vi "Extract Video Moments.vi"() -> ()   [LabVIEW 2026]
uses:
  90f86d5b-f17d-465b-a039-599a13c3f885.vi
panel:
  out "Web Browser Control":string(html)
  out "appended array":cluster{"output 7":dbl, "Instruction":string}[](array[cluster])
  in  "Video to Inject":path=path "C:/ProgramData/LabVIEWEval/Protected/19 - Block Diagram Demonstration Summary.mp4"
  in  "stop":bool
  in  "Create Marker":bool
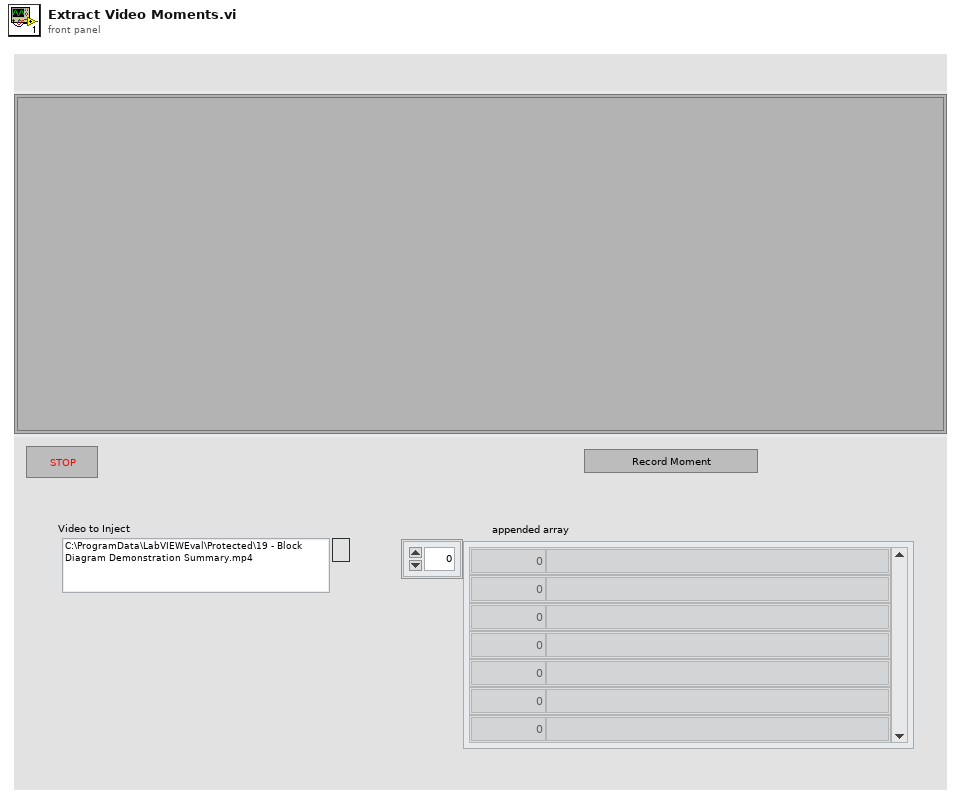
[diagram p1: front panel]
types:
  T1 = enum16{"open", "replace", "create", "open or create", "replace or create", "replace or create with confirmation"}
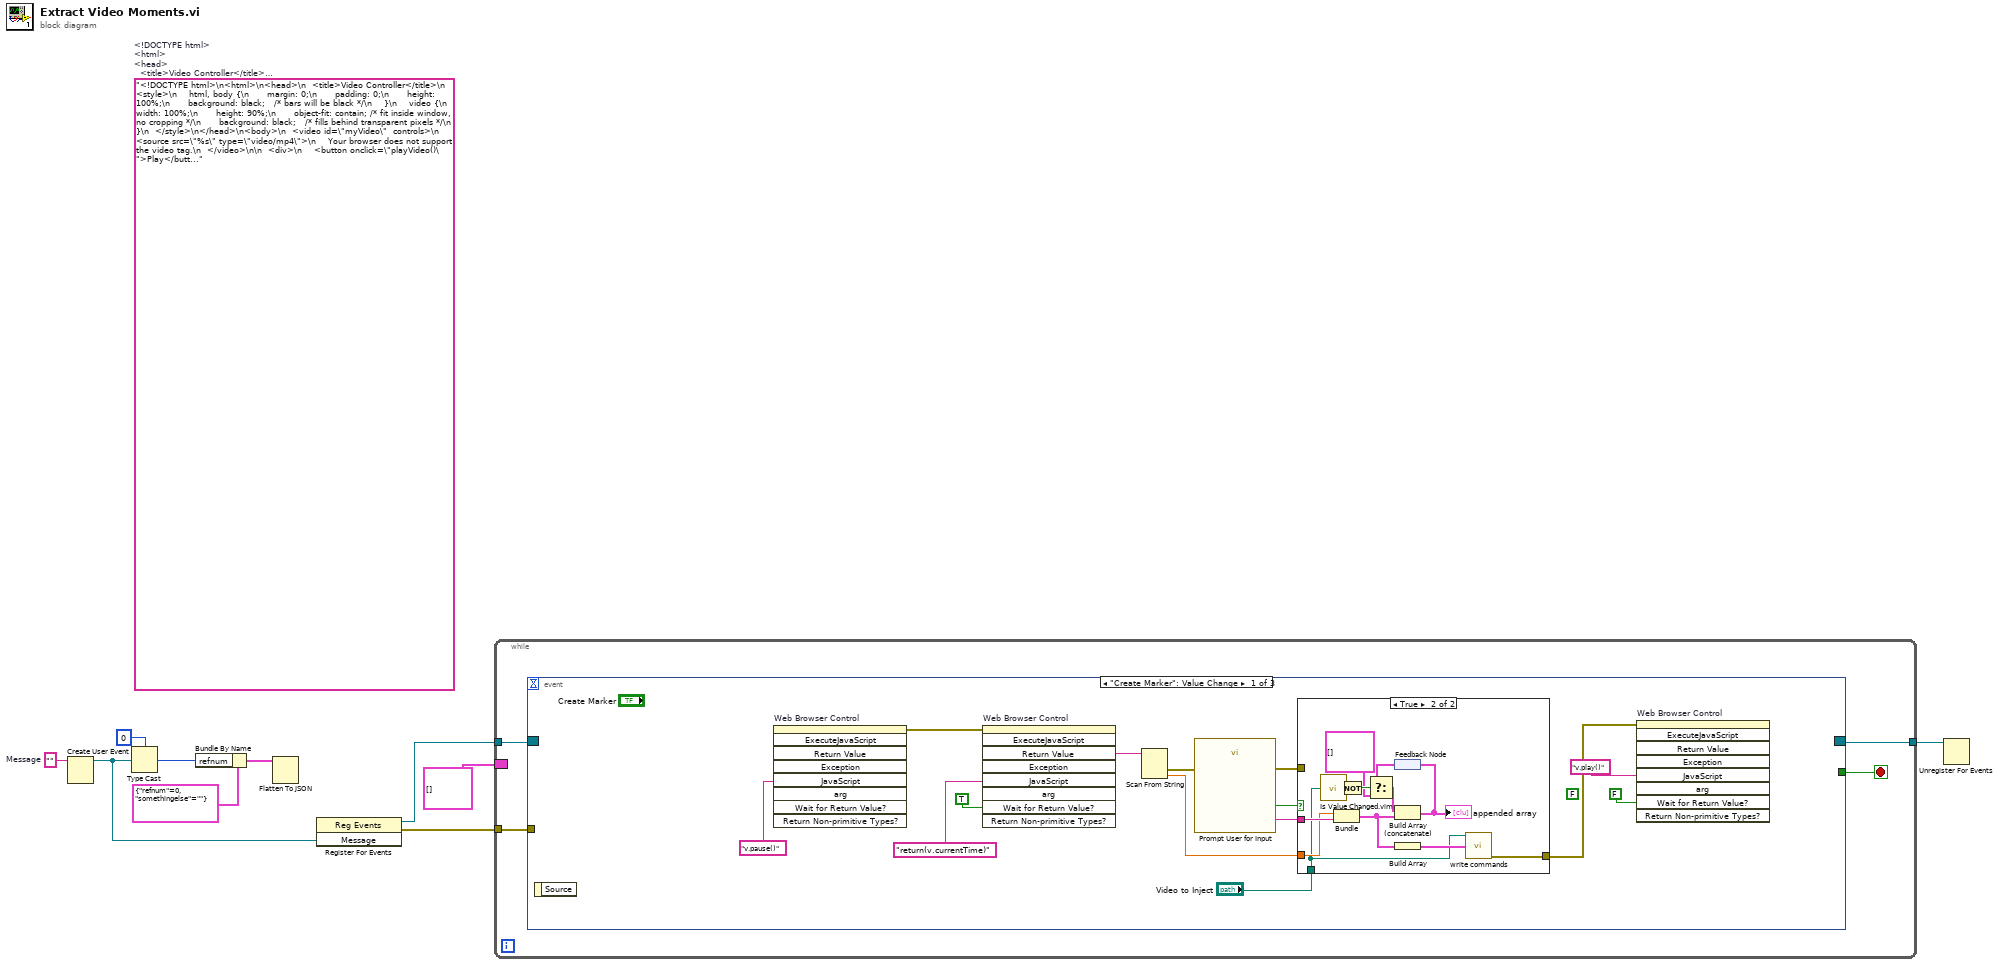
[diagram p0: block diagram]
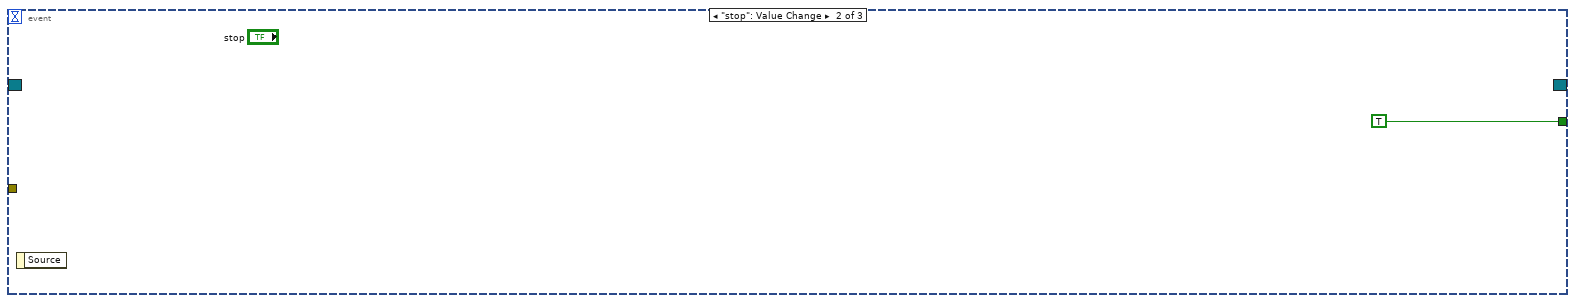
[diagram p3: hidden frame]
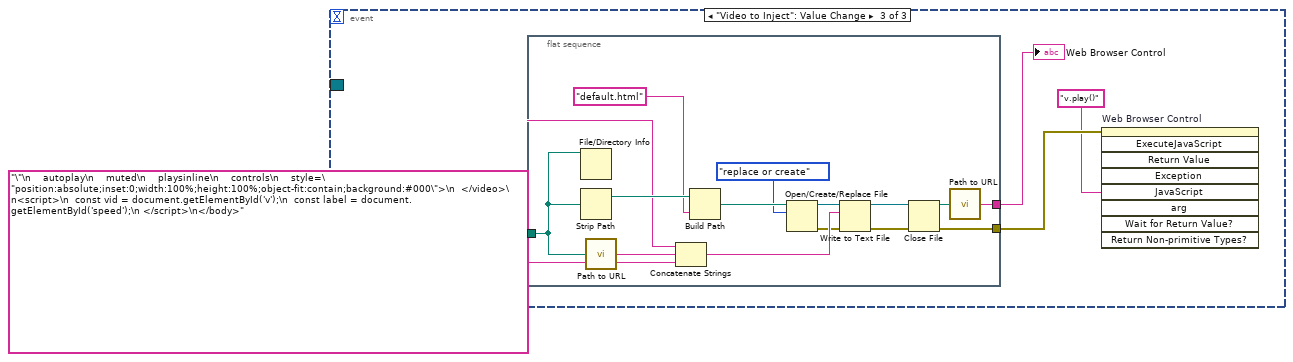
[diagram p4: hidden frame]
diagram:
  w2 = ""  # Message
  (unwired) "<!DOCTYPE html>\n<html>\n<head>\n  <title>Video Controller</title>\n  <style>\n    html, body {\n      margin: 0;\n      padding: 0;\n      height: 100%;\n      background: black;   /* bars will be black */\n    }\n    video {\n      width: 100%;\n      height: 90%;\n      object-fit: contain; /* fit inside window, no cropping */\n      background: black;   /* fills behind transparent pixels */\n    }\n  </style>\n</head>\n<body>\n  <video id=\"myVideo\"  controls>\n    <source src=\"%s\" type=\"video/mp4\">\n    Your browser does not support the video tag.\n  </video>\n\n  <div>\n    <button onclick=\"playVideo()\">Play</button>\n    <button onclick=\"pauseVideo()\">Pause</button>\n    <button onclick=\"rewindVideo()\">Rewind 5s</button>\n    <button onclick=\"skipVideo()\">Skip 5s</button>\n    <button onclick=\"changeSpeed()\">Toggle Speed</button>\n  </div>\n\n    <script>\n    const video = document.getElementById('myVideo');\n    let fast = false;\n\n    function playVideo() {\n      video.play();\n    }\n\n    function pauseVideo() {\n      video.pause();\n    }\n\n    function rewindVideo() {\n      video.currentTime -= 5;\n    }\n\n    function skipVideo() {\n      video.currentTime += 5;\n    }\n\n    function changeSpeed() {\n      video.playbackRate = fast ? 1.0 : 2.0;\n      fast = !fast;\n    }\n\n    // Example: detect when the video ends\n    video.onended = () => {\n      //alert(\"Video has finished playing.\");\n    }\n\n    let fired = false; // make sure we only fire once\n\n    video.addEventListener('timeupdate', () => {\n      if (!fired && video.currentTime >= 10) {\n        fired = true;\n        //alert(\"Reached 10 seconds!\");\n        // Dispatch a custom event\n\n      }\n    });\n  function getCurrentVideoTime() {\n    const v = document.querySelector('video');\n    if (!v) {\n      console.warn(\"No <video> element found.\");\n      return null;\n    }\n    return v.currentTime;  // returns time in seconds (float)\n  }\n\n  // Example: log current time whenever you click the page\n  document.addEventListener('click', () => {\n    console.log(\"Video current time:\", getCurrentVideoTime());\n  });\n  </script>\n</body>\n</html>\n"  # <!DOCTYPE html> <html> <head>   <title>Video Controller</title>   <style>     html, body {       margin: 0;       padding: 0;       height: 100%;       background: black;   /* bars will be black */     }     video {       width: 100%;       height: 90%;       object-fit: contain; /* fit inside window, no cropping */       background: black;   /* fills behind transparent pixels */     }   </style> </head> <body>   <video id="myVideo"  controls>     <source src="%s" type="video/mp4">     Your browser does not support the video tag.   </video>    <div>     <button onclick="playVideo()">Play</button>     <button onclick="pauseVideo()">Pause</button>     <button onclick="rewindVideo()">Rewind 5s</button>     <button onclick="skipVideo()">Skip 5s</button>     <button onclick="changeSpeed()">Toggle Speed</button>   </div>      <script>     const video = document.getElementById('myVideo');     let fast = false;      function playVideo() {       video.play();     }      function pauseVideo() {       video.pause();     }      function rewindVideo() {       video.currentTime -= 5;     }      function skipVideo() {       video.currentTime += 5;     }      function changeSpeed() {       video.playbackRate = fast ? 1.0 : 2.0;       fast = !fast;     }      // Example: detect when the video ends     video.onended = () => {       //alert("Video has finished playing.");     }      let fired = false; // make sure we only fire once      video.addEventListener('timeupdate', () => {       if (!fired && video.currentTime >= 10) {         fired = true;         //alert("Reached 10 seconds!");         // Dispatch a custom event        }     });   function getCurrentVideoTime() {     const v = document.querySelector('video');     if (!v) {       console.warn("No <video> element found.");       return null;     }     return v.currentTime;  // returns time in seconds (float)   }    // Example: log current time whenever you click the page   document.addEventListener('click', () => {     console.log("Video current time:", getCurrentVideoTime());   });   </script> </body> </html>
  n1 = Create User Event(user event datatype=w2) -> (user event=w1:refnum<user-event>)  [unwired: 1 in, 1 out]
  n2 = Type Cast(type=u32 0, x=w1) -> (*(type *) &x=w6:u32)
  n3 = Bundle By Name(cluster=cluster{"refnum":u32, "somethingelse":string} {"refnum"=0, "somethingelse"=""}, "refnum"=w6) -> (w4:cluster{"refnum":u32, "somethingelse":string})
  n4 = Flatten To JSON(anything=w4) -> ()  [unwired: 2 in, 2 out]
  n5 = register-events(w1) -> (reference out=w10:refnum<event-registration>, error out=w9:errorcluster)  [unwired: 2 in]
  n6 = while {
    tunnel: w10 -> [w12]
    tunnel: w9 -> [w13]
    tunnel: [w11] -> w8
    border: cluster{"output 7":dbl, "Instruction":string}[] [] -> [_]
    stop <- w14 stop-if-true
    n7 = event shown="[0] \"Create Marker\": Value Change" {
      selector: w12 -> [_ _ _]
      dyn-events: [_ _ _] -> w11
      timeout: _ -> [_ _ _]
      tunnel: [_ TRUE _] -> w14
      tunnel: w13 -> [_ _ _]
      event "Create Marker": Value Change {
        (unwired) FALSE ("Decode Result")
        n8 = event-data() -> ()  [unwired: 1 in, 1 out]
        n9 = invoke on="Web Browser Control" class="WebBrowser (strict)" method="ExecuteJavaScript"("JavaScript"="v.pause()" ("javaScript")) -> (error out=w23:errorcluster)  [unwired: 8 in, 8 out]
        n10 = invoke on="Web Browser Control" class="WebBrowser (strict)" method="ExecuteJavaScript"(error in=w23, "JavaScript"="return(v.currentTime)" ("javaScript"), "Wait for Return Value?"=TRUE ("Fetch Result")) -> ("Return Value"=w20:string)  [unwired: 6 in, 8 out]
        n11 = Scan From String(input string=w20) -> (error out=w26:errorcluster, output 1=w27:dbl)  [unwired: 4 in, 2 out]
        n12 = call "Prompt User for Input"("error in (no error)"=w26) -> ("Instruction"=w28:string, "OK"=w25:bool, "error out"=w16:errorcluster)  [unwired: 16 in]
        n13 = case shown="True" w25 {
          tunnel: w28 -> [_ w41]
          tunnel: w27 -> [_ w40]
          tunnel: "Video to Inject" -> [_ w35]
          tunnel: [w29 w30] -> w17
          tunnel: w16 -> [w29 _]
          frame False {
          }
          frame True {
            n14 = call "Is Value Changed.vim"("value"=w35) -> ("changed or first call?"=w34:bool)
            n15 = Bundle(w40, "Instruction"=w41) -> (w37:cluster{dbl, "Instruction":string})  [unwired: 1 in]
            n16 = Not(x=w34) -> (.not. x?=w32:bool)
            n17 = feedback #1() -> (w39:cluster{"output 7":dbl, "Instruction":string}[])
            n18 = Select(t=w39, s=w32, f=cluster{dbl, "Instruction":string}[] []) -> (s? t:f=w33:cluster{"output 7":dbl, "Instruction":string}[])
            n19 = Build Array (concatenate)(w33, w37) -> (w38:cluster{"output 7":dbl, "Instruction":string}[])
            "appended array" <- w38
            n20 = feedback-in #1(w38) -> ()
            n21 = Build Array(w37) -> (w36:cluster{dbl, "Instruction":string}[])
            n22 = call "write commands.vi"("Video to Inject"=w35, "Commands"=w36) -> ("error out"=w30:errorcluster)  [unwired: 13 in]
          }
        }
        n23 = invoke on="Web Browser Control" class="WebBrowser (strict)" method="ExecuteJavaScript"(error in=w17, "JavaScript"="v.play()" ("javaScript"), "Wait for Return Value?"=FALSE ("Fetch Result")) -> ()  [unwired: 6 in, 9 out]
      }
      event "stop": Value Change {
        n24 = event-data() -> ()  [unwired: 1 in, 1 out]
      }
      event "Video to Inject": Value Change {
        n25 = event-data() -> ("NewVal"=w46:path)  [unwired: 1 in]
        n26 = flat-sequence {
          tunnel: w46 -> [w54]
          tunnel: [w53] -> w45
          tunnel: [w47] -> w44
          frame #0 {
            # "`"
            n27 = File/Directory Info(path=w54) -> ()  [unwired: 1 in, 7 out]
            n28 = Strip Path(path=w54) -> (stripped path=w62:path)  [unwired: 1 out]
            n29 = call <vilib>:"Path to URL.vi"("path"=w54) -> ("url"=w61:string)
            n30 = Concatenate Strings("<!DOCTYPE html>\n<body>\n  <video\nid=\"v\"\n    src=\"", w61, "\"\n    autoplay\n    muted\n    playsinline\n    controls\n    style=\"position:absolute;inset:0;width:100%;height:100%;object-fit:contain;background:#000\">\n  </video>\n<script>\n  const vid = document.getElementById('v');\n  const label = document.getElementById('speed');\n </script>\n</body>") -> (w55:string)
            n31 = Build Path(base path=w62, name or relative path="default.html") -> (appended path=w51:path)
            n32 = Open/Create/Replace File(file path (use dialog)=w51, operation (0:open)=T1."replace or create") -> (refnum out=w50:refnum<file>, error out=w52:errorcluster)  [unwired: 4 in, 1 out]
            n33 = Write to Text File(file (use dialog)=w50, text=w55, error in=w52) -> (refnum out=w59:refnum<file>, error out=w60:errorcluster)  [unwired: 1 in, 1 out]
            n34 = Close File(refnum=w59, error in=w60) -> (path=w58:path, error out=w47:errorcluster)
            n35 = call <vilib>:"Path to URL.vi"("path"=w58) -> ("url"=w53:string)
          }
        }
        n36 = invoke on="Web Browser Control" class="WebBrowser (strict)" method="ExecuteJavaScript"(error in=w44, "JavaScript"="v.play()" ("javaScript")) -> ()  [unwired: 7 in, 9 out]
        "Web Browser Control" <- w45
      }
    }
  }
  n37 = Unregister For Events(event registration refnum=w8) -> ()  [unwired: 1 in, 1 out]
